vi "Keithley_ConfirmJump.vi"(0 "VISA resource name in":refnum<visa-resource-name>, 3 "error in":errorcluster, 4 "Gate Voltage\nInitial (V)":dbl) -> (7 "VISA resource name out":refnum<visa-resource-name>, 8 "Voltage OK?":bool, 10 "error out":errorcluster)   [LabVIEW 2021]
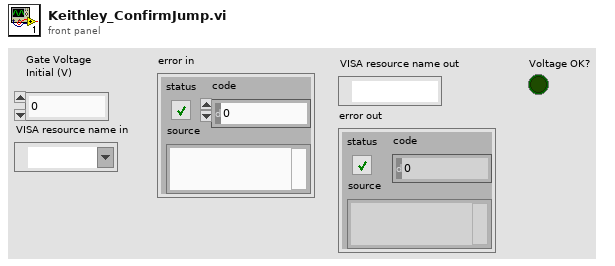
[diagram p1: front panel]
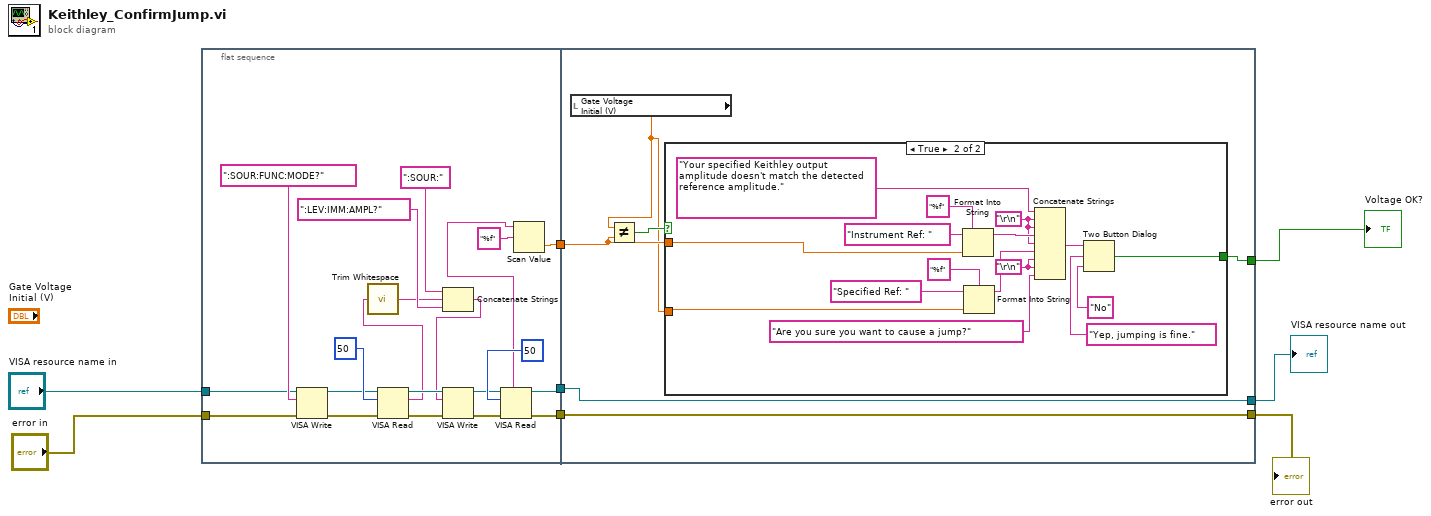
[diagram p0: block diagram]
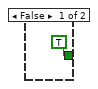
[diagram p2: hidden frame]
diagram:
  n1 = flat-sequence {
    tunnel: [w11] -> w8
    tunnel: [w12] -> w7
    tunnel: [w13] -> w6
    tunnel: "VISA resource name in" -> [w10]
    tunnel: "error in" -> [w9]
    tunnel: w8 -> [w32]
    tunnel: w7 -> [w31]
    tunnel: w6 -> [w35]
    tunnel: [w32] -> w3
    tunnel: [w31] -> w2
    tunnel: [w30] -> w1
    frame #0 {
      n2 = VISA Write(VISA resource name=w10, write buffer=":SOUR:FUNC:MODE?", error in (no error)=w9) -> (VISA resource name out=w26:refnum<visa-resource-name>, error out=w29:errorcluster)  [unwired: 1 out]
      n3 = VISA Read(VISA resource name=w26, byte count=u32 50, error in (no error)=w29) -> (VISA resource name out=w21:refnum<visa-resource-name>, read buffer=w15:string, error out=w22:errorcluster)  [unwired: 1 out]
      n4 = call <vilib>:"Trim Whitespace.vi"("string"=w15) -> ("trimmed string"=w14:string)  [unwired: 1 in]
      n5 = Concatenate Strings(":SOUR:" ("string"), w14, ":LEV:IMM:AMPL?" ("string")) -> (w18:string)
      n6 = VISA Write(VISA resource name=w21, write buffer=w18, error in (no error)=w22) -> (VISA resource name out=w23:refnum<visa-resource-name>, error out=w25:errorcluster)  [unwired: 1 out]
      n7 = VISA Read(VISA resource name=w23, byte count=u32 50, error in (no error)=w25) -> (VISA resource name out=w11:refnum<visa-resource-name>, read buffer=w16:string, error out=w12:errorcluster)  [unwired: 1 out]
      n8 = Scan Value(string=w16, format string="%f") -> (value=w13:dbl)  [unwired: 1 in, 1 out]
    }
    frame #1 {
      n9 = local read "Gate Voltage\nInitial (V)"() -> (w33:dbl)
      n10 = Not Equal?(x=w33, y=w35) -> (x != y?=w34:bool)
      n11 = case shown="True" w34 {
        tunnel: [TRUE ("T button?") w43] -> w30
        tunnel: w35 -> [_ w38]
        tunnel: w33 -> [_ w37]
        frame False {
        }
        frame True {
          w41 = "\r\n"
          w39 = "\r\n"
          n12 = Format Into String(format string="%f", initial string="Instrument Ref: ", w38) -> (resulting string=w45:string)  [unwired: 1 in, 1 out]
          n13 = Format Into String(format string="%f", initial string="Specified Ref: ", w37) -> (resulting string=w44:string)  [unwired: 1 in, 1 out]
          n14 = Concatenate Strings("Your specified Keithley output amplitude doesn't match the detected reference amplitude." ("message"), w39, w39, w45, w39, w44, w41, w41, "Are you sure you want to cause a jump?" ("string")) -> (w50:string)
          n15 = Two Button Dialog(message=w50, 1:"No" ("F button name (\"Cancel\")"), 2:"Yep, jumping is fine." ("T button name (\"OK\")")) -> (T button?=w43:bool)
        }
      }
    }
  }
  "VISA resource name out" <- w3
  "error out" <- w2
  "Voltage OK?" <- w1
